vi "ADC Data capture and Process Original.vi"(0 "ADC Output Read Method":T2(ring)=enum."Read .dat file", 1 "Select the Tab to project":T1(ring)=enum."ADC Sine", 2 "ADC Input":enum16{"Sine Wave", "Ramp / Triangle"}(ring), 3 "No.of samples(SNR)":i32=4096, 4 "Resolution":i32=12, 5 "active edge":i32(ring)=10280, 6 "Inputs for Dyanmic para":T9={"Fundamental Frequency"=100000.0, "Sampling Frequncy"=3999610.0, "No of Harmonics"=9, "Window"=enum."7 Term B-Harris", "Blackman (fundamental power) bins)"=1.0}, 7 "Samples per Channel":i32=4096 caption="No.of Samples(capture)", 8 "Oversampling":bool, 9 "Oversampling ratio":i32, 10 "Drop LSB":bool, 11 "Save data":T15, 12 "Waveform":i64[](array[numeric]), 13 "Path to Read":path=path "C/Users/a0230227/Desktop/save.dat", 14 "Start & Stop Bit":cluster{"Start":i32, "Stop":i32}={"Start"=40, "Stop"=4055}, 15 "length":i32=4096, 17 "Set_Freq":dbl=100017.0, 24 "path to save":T14={"Path to Save plot"=path "D/Tenor_176P/DYN_PAR_C004/DAT/D001_TEMPP30C_VDD1.2_VDDA3.3_16B_SE_ADCA__vicA_aggX_PLT_CAP_200821_1740_33.jpg", "Path to Raw Data plot"=path "D/Tenor_176P/DYN_PAR_C004/DAT/D001_TEMPP30C_VDD1.2_VDDA3.3_16B_SE_ADCA__vicA_aggX_RAW_DAT_200821_1740_33.csv"}) -> (18 "Min Max":T4, 19 "detected Throughput":dbl, 20 "output cluster":T7, 21 "Dynamic Parameters":T8, 22 "max code":ext, 23 "min code":ext, 25 "Valid Capture":bool)   [LabVIEW 2021] (continued)
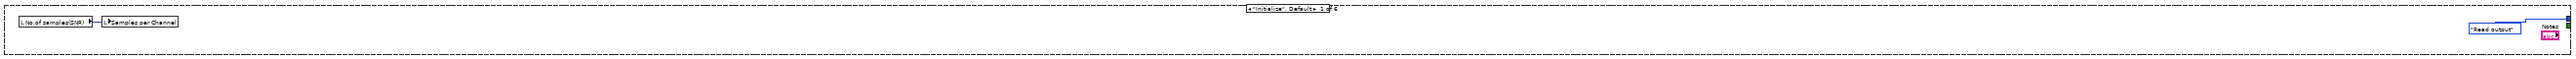
[diagram p2: hidden frame]
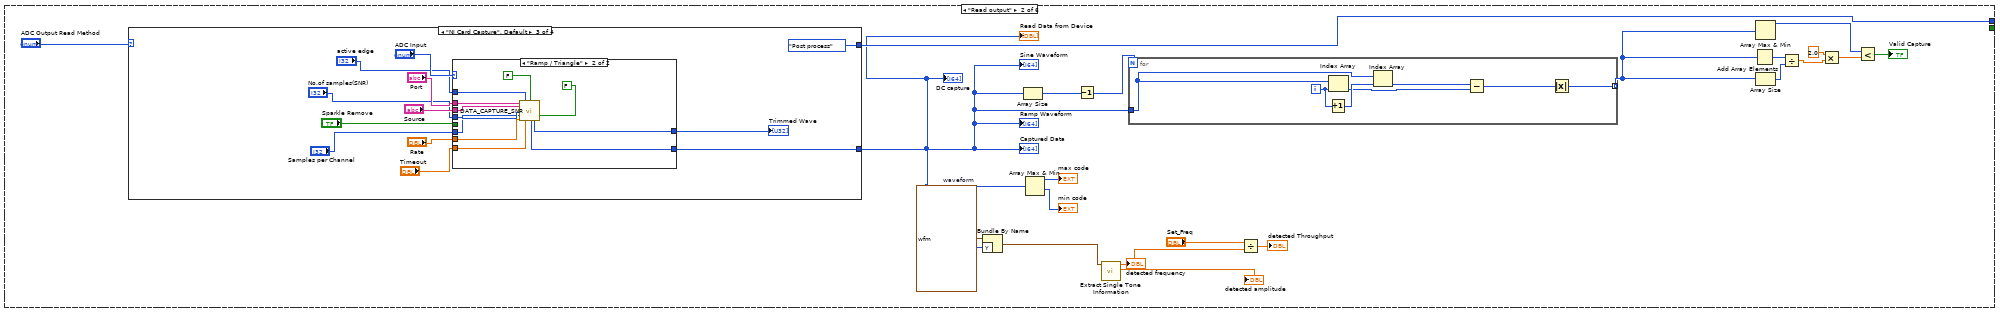
[diagram p3: hidden frame]
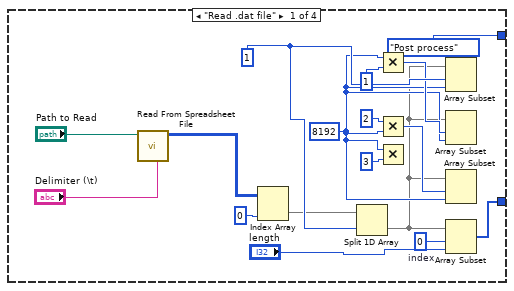
[diagram p4: hidden frame]
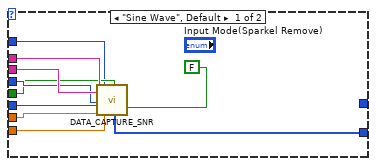
[diagram p6: hidden frame]
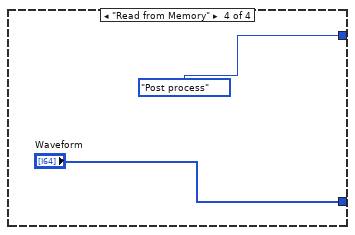
[diagram p7: hidden frame]
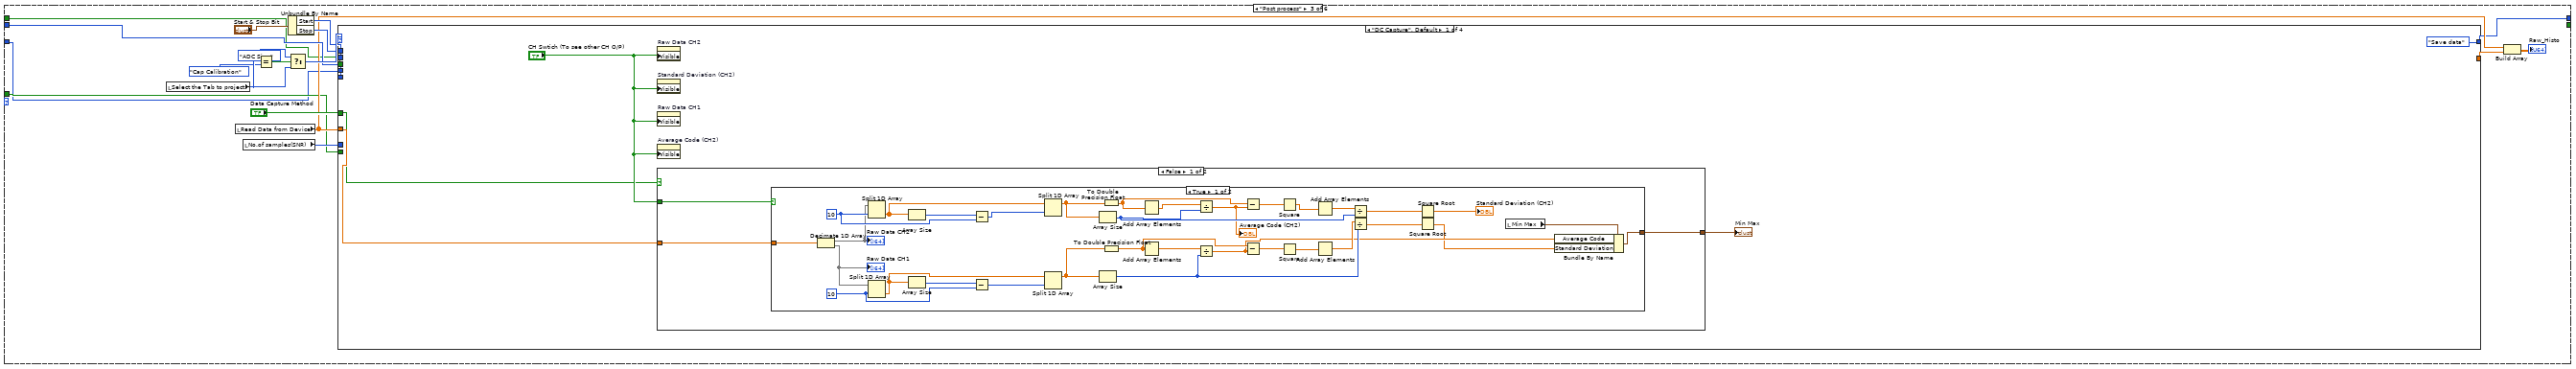
[diagram p8: hidden frame]
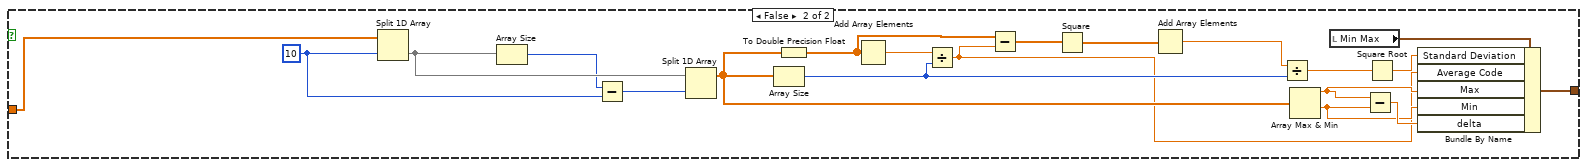
[diagram p9: hidden frame]
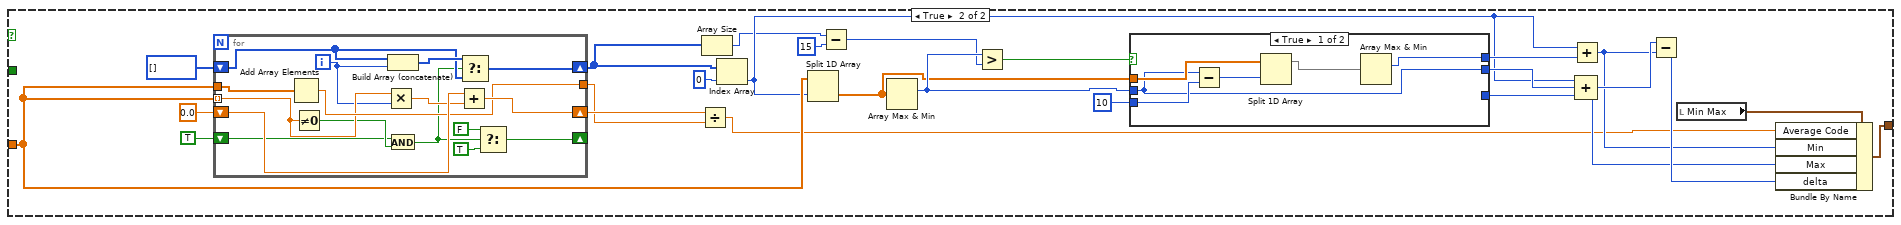
[diagram p10: hidden frame]
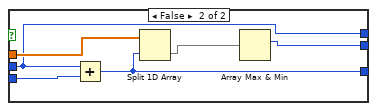
[diagram p11: hidden frame]
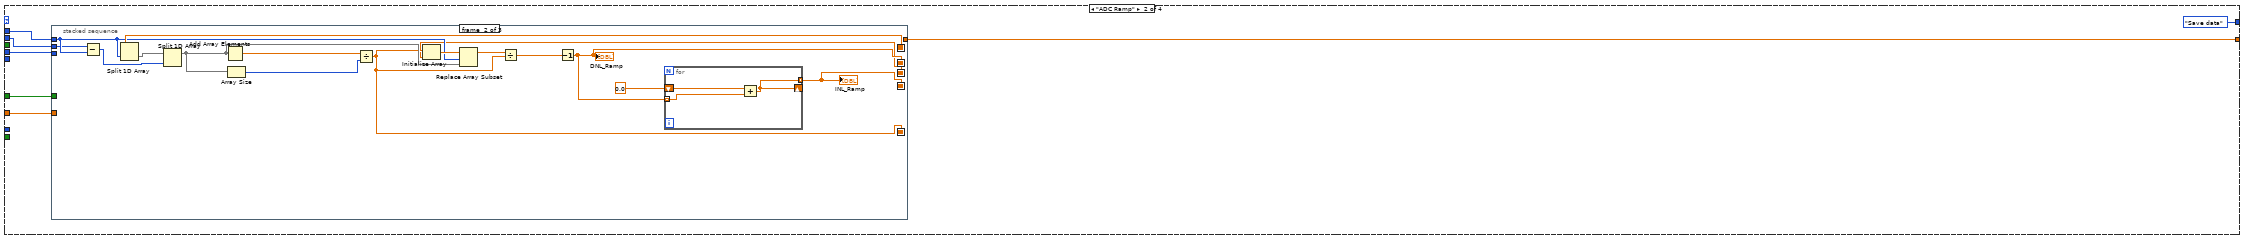
[diagram p12: hidden frame]
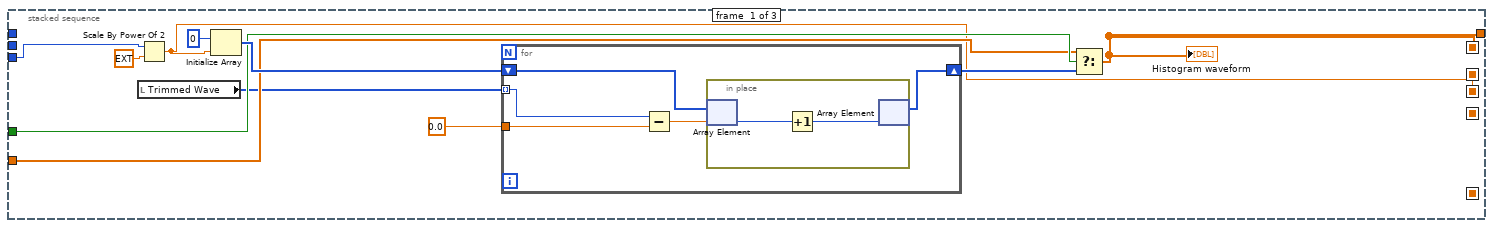
[diagram p13: hidden frame]
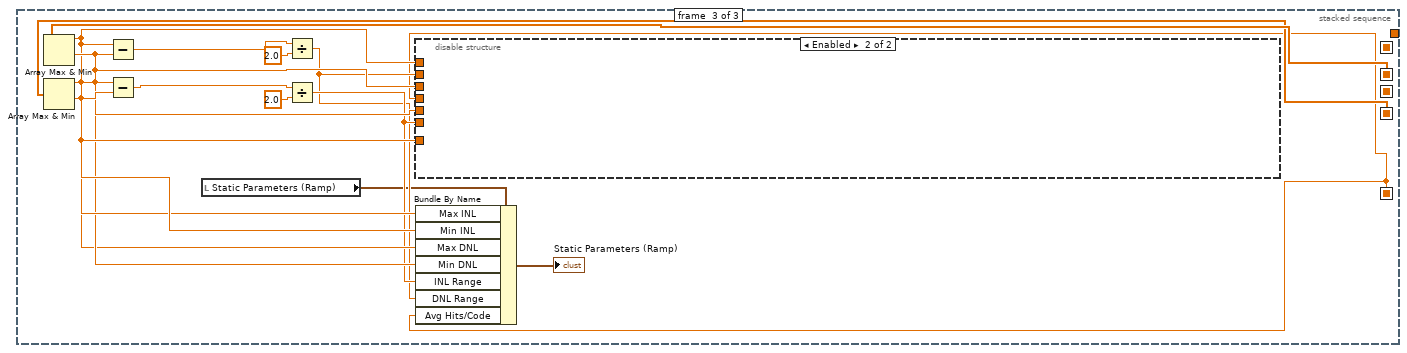
[diagram p14: hidden frame]
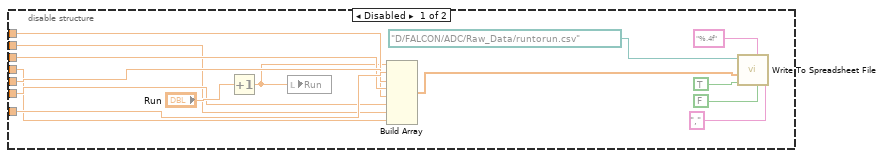
[diagram p15: hidden frame]
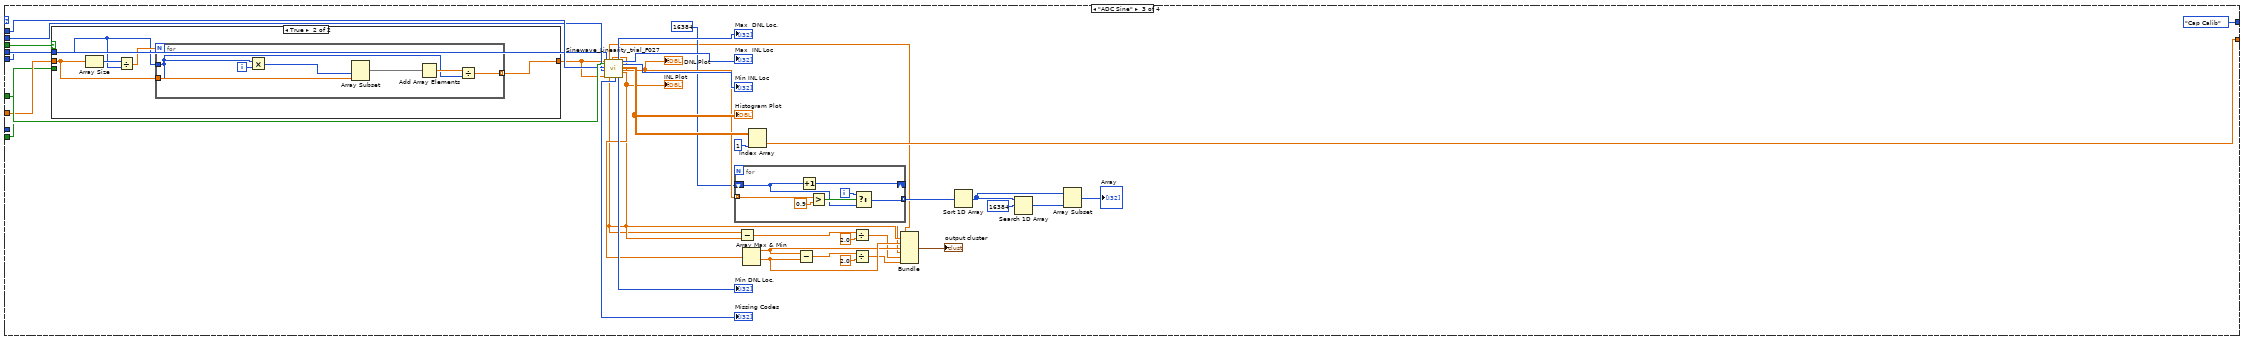
[diagram p16: hidden frame]
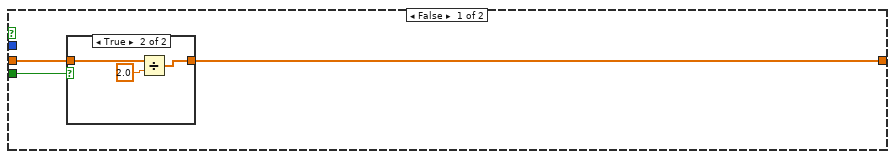
[diagram p17: hidden frame]
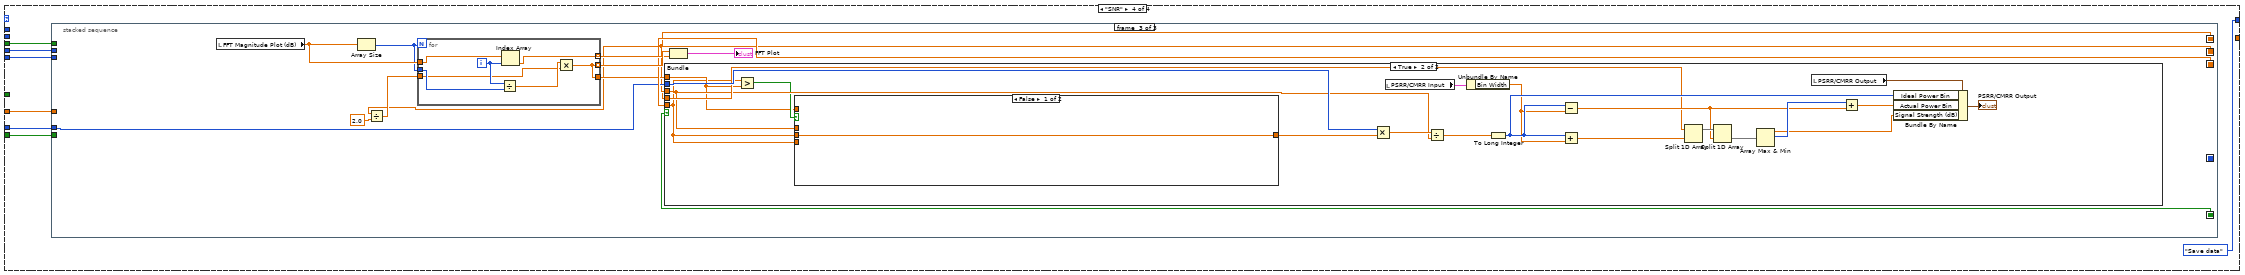
[diagram p19: hidden frame]
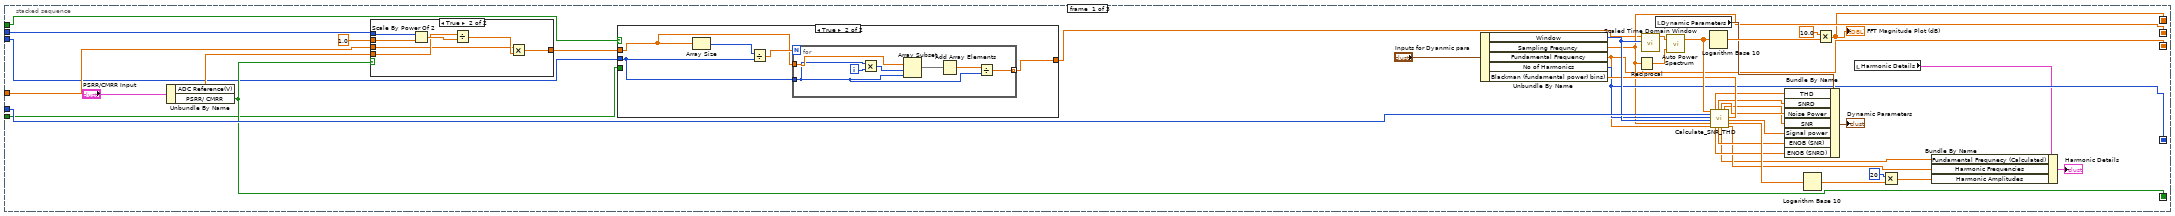
[diagram p20: hidden frame]
                n298 = call "Take fron panel screenshot.vi"("VI path"=w619, "Image path"=w618, "Visible area only? (f)"=FALSE, "File type (.jpg)"=enum16{".bmp", ".png", ".jpg"}.".png") -> ()  [unwired: 4 in, 1 out]
              }
            }
            n299 = case shown="True" w612 {
              tunnel: w615 -> [_ w624]
              frame False {
              }
              frame True {
                n300 = local read "FFT Plot"() -> (w629:cluster{dbl[], dbl[]})
                n301 = local read "Captured Data"() -> (w628:i64[])
                n302 = Unbundle(w629) -> (w627:dbl[], w626:dbl[])
                n303 = Build Array(w628, w627, w626) -> (w625:dbl[][])
                n304 = call-poly <vilib>:"Write To Spreadsheet File.vi"("delimiter (\\t)"="," ("delimiter (\\t)"), "transpose? (no:F)"=TRUE, "2D data"=w625, "file path (dialog if empty)"=w624) -> ()  [unwired: 4 in, 1 out]
              }
            }
            n305 = local write "Main Tab"(5) -> ()
            "SNR" <- 2
          }
          frame "Cap Calibration" {
            n306 = local write "Main Tab"(6) -> ()
          }
          frame "DC Capture" {
            n307 = case shown="True" w631 {
              tunnel: w632 -> [_ w637]
              frame False {
              }
              frame True {
                n308 = local read "DC capture"() -> (w634:i64[])
                n309 = call-poly <vilib>:"Write To Spreadsheet File.vi"("delimiter (\\t)"="" ("delimiter (\\t)"), "transpose? (no:F)"=TRUE, "1D data"=w634, "file path (dialog if empty)"=w637) -> ()  [unwired: 4 in, 1 out]
              }
            }
            n310 = local write "Main Tab"(2) -> ()
          }
        }
      }
      frame "Exit" {
        n311 = disable-structure shown="Enabled" {
          frame Enabled {
            w639 = FALSE ("Save INL/DNL Plot(Ramp)")
            n312 = local read "Save data"() -> (w641:T15)
            n313 = Bundle By Name(cluster=w641, "Save INL/DNL Plot(Ramp)"=w639, "Save SNR Plot"=w639, "Save INL/DNL Plot(Sine)"=w639, "Save INL/DNL Raw Data(Ramp)"=w639, "Save SNR Raw Data"=w639, "Save INL/DNL Raw Data(Sine)"=w639, "Save  Raw Data(Sine)"=w639) -> (w640:T15)
            n314 = local write "Save data"(w640) -> ()
          }
          frame Disabled {
          }
        }
        n315 = disable-structure shown="Disabled" {
          frame Disabled {
            n316 = local write item#-1(u32 12000 ("Wait time to Read Memory \n(To complete Conv) mS")) -> ()
          }
          frame Enabled {
          }
        }
      }
    }
  }
